vi "Add Barista.vi"(7 "Time Scale [ms]":u32=7000, 8 "error in (no error)":errorcluster, 10 "Name":string, 11 "Coffee Shop in":refnum<class "Coffee Shop.lvclass">) -> (0 "error out":errorcluster, 3 "Coffee Shop out":refnum<class "Coffee Shop.lvclass">)   [LabVIEW 2020, in "Coffee Shop.lvclass"]
uses:
  Coffee Shop.lvclass
  C:/Program Files (x86)/National Instruments/LabVIEW 2020/vi.lib/Astemes/Triarc Framework/Process/Process.lvclass
  People/Workers/Barista/Barista.lvclass
  C:/Git/astemes-triarc-examples/Coffee Shop/Processes/People/Person/Person.lvclass
  People/Person/Person.lvclass/Person.ctl
  <vilib>/Astemes/Triarc Framework/Process/Process.lvclass/Process.ctl
  <vilib>/Astemes/Triarc Framework/Process/Public/Lifecycle/Get Lifecycle State.vi
  <vilib>/Astemes/Triarc Framework/Process/Private/SubVIs/Handle Debug Data.vi
  <vilib>/Utility/error.llb/Clear Errors.vi
  <vilib>/Astemes/Triarc Framework/Logging/Log Debug.vi
  <vilib>/AdvancedString/1D String Array to Delimited String.vi
  <vilib>/Utility/High Resolution Relative Seconds.vi
  <vilib>/Utility/error.llb/Error Cluster From Error Code.vi
  <vilib>/Astemes/Triarc Framework/Process/Public/Read Name.vi
  Coffee Shop.lvclass/Coffee Shop.ctl
  People/Person/Person.lvclass
  <vilib>/Astemes/Triarc Framework/Process/Process.lvclass
  C:/Git/astemes-triarc-examples/Coffee Shop/Processes/People/Workers/Worker/Worker.lvclass
  C:/Program Files (x86)/National Instruments/LabVIEW 2020/vi.lib/Astemes/Triarc Framework/View/View.lvclass
  C:/Program Files (x86)/National Instruments/LabVIEW 2020/vi.lib/Astemes/Triarc Framework/Base/Base.lvclass
  C:/Program Files (x86)/National Instruments/LabVIEW 2020/vi.lib/Astemes/Triarc Framework/Error Handler Interface/Error Handler Interface.lvclass
  C:/Program Files (x86)/National Instruments/LabVIEW 2020/vi.lib/Astemes/Triarc Framework/Logging/Logging.lvclass
  C:/Git/astemes-triarc-examples/Coffee Shop/Processes/People/Process Job/Job Handler.lvclass
  C:/Git/astemes-triarc-examples/Coffee Shop/Processes/People/Workers/Barista/Barista.lvclass
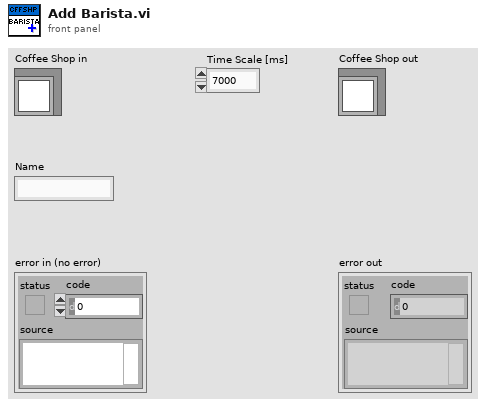
[diagram p1: front panel]
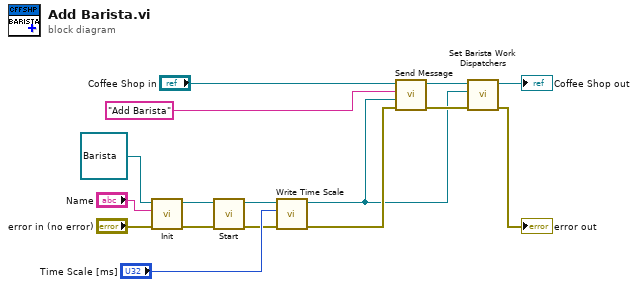
[diagram p0: block diagram]
diagram:
  n1 = call-dynamic "Init.vi"("error in (no error)"="error in (no error)", "Name"="Name", "View In"=refnum<class "Barista.lvclass"> refnum ("Barista.lvclass")) -> ("error out"=w10:errorcluster, "View Out"=w2:refnum<class "Barista.lvclass">)  [unwired: 7 in]
  n2 = call <vilib>:"Start.vi"("error in (no error)"=w10, "Process In"=w2) -> ("error out"=w3:errorcluster, "Process Out"=w1:refnum<class "Barista.lvclass">)  [unwired: 7 in, 1 out]
  n3 = call "Write Time Scale.vi"("error in (no error)"=w3, "Time Scale [ms]"="Time Scale [ms]", "Person In"=w1) -> ("error out"=w6:errorcluster, "Person In"=w5:refnum<class "Barista.lvclass">)  [unwired: 7 in]
  n4 = call <vilib>:"Send Message.vi"("error in (no error)"=w6, "Message Data"=w5, "Message"="Add Barista", "Process In"="Coffee Shop in") -> ("error out"=w16:errorcluster, "Process Out"=w8:refnum<class "Coffee Shop.lvclass">)  [unwired: 6 in]
  n5 = call "Set Barista Work Dispatchers.vi"("error in (no error)"=w16, "Barista"=w5, "Coffee Shop In"=w8) -> ("error out"=→"error out":errorcluster, "Coffee Shop Out"=→"Coffee Shop out":refnum<class "Coffee Shop.lvclass">)  [unwired: 7 in]
